vi "Open or Create.vi"(8 "error in":errorcluster, 9 "SheetName":string="Sheet1", 10 "Path":path) -> (0 "error out":errorcluster, 3 "SpreadsheetDoc":refnum<k24>)   [LabVIEW 2019, in "Open Xml.lvlib"]
uses:
  Open Xml.lvlib
  D:/git/Open-Xml-LabVIEW/Source/DocumentFormat.OpenXml.dll
  DocumentFormat.OpenXml.dll
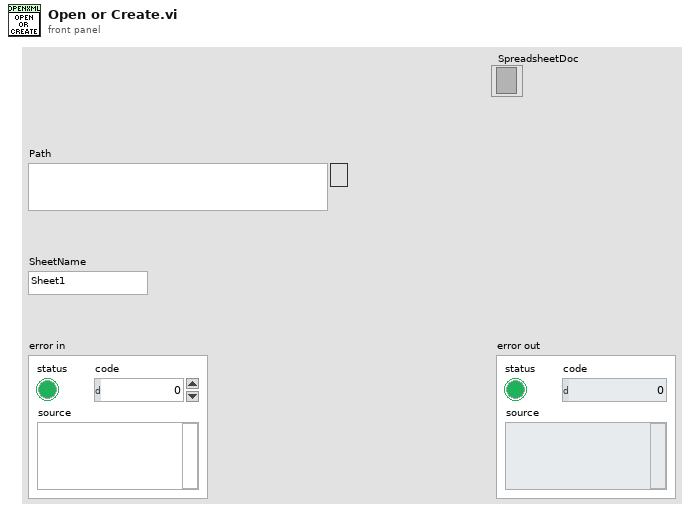
[diagram p1: front panel]
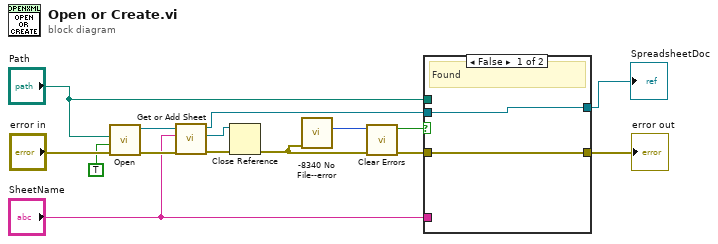
[diagram p0: block diagram]
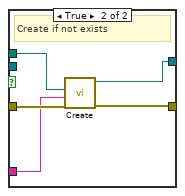
[diagram p2: hidden frame]
diagram:
  n1 = call "Open.vi"("error in"="error in", "isEditable"=TRUE, "Path"="Path") -> ("error out"=w7:errorcluster, "SpreadsheetDoc"=w5:refnum<k24>)  [unwired: 7 in]
  n2 = call "Get or Add Sheet.vi"("error in"=w7, "Sheet Name"="SheetName", "SpreadsheetDoc in"=w5) -> ("error out"=w4:errorcluster, "Sheet"=w1:refnum<k24>, "SpreadsheetDoc out"=w3:refnum<k24>)  [unwired: 5 in, 1 out]
  n3 = Close Reference(reference=w1, error in (no error)=w4) -> (error out=w2:errorcluster)
  n4 = call "-8340 No File--error.vi"("error in (no error)"=w2) -> ("Error Code"=w14:i32)  [unwired: 9 in, 1 out]
  n5 = call <vilib>:"Clear Errors.vi"("error in (no error)"=w2, "specific error code to clear (0: all)"=w14) -> ("error out"=w15:errorcluster, "specific error cleared?"=w12:bool)  [unwired: 4 in]
  n6 = case shown="False" w12 {
    tunnel: w15 -> [w17 w22]
    tunnel: "SheetName" -> [_ w21]
    tunnel: [w17 w18] -> w10
    tunnel: w3 -> [w16 _]
    tunnel: [w16 w19] -> w11
    tunnel: "Path" -> [_ w20]
    frame False {
      # "Found"
    }
    frame True {
      # "Create if not exists"
      n7 = call "Create.vi"("error in"=w22, "SheetName"=w21, "Path"=w20) -> ("error out"=w18:errorcluster, "SpreadsheetDoc"=w19:refnum<k24>)  [unwired: 7 in]
    }
  }
  "SpreadsheetDoc" <- w11
  "error out" <- w10
